vi "Limit ILC Voltage.vi"(8 "error in (no error)":errorcluster, 10 "Voltage in":dbl[unit], 11 "Limit ILC Voltage in":refnum<class "Limit ILC Voltage.lvclass">) -> (0 "error out":errorcluster, 2 "Voltage out":dbl[unit], 3 "Limit ILC Voltage out":refnum<class "Limit ILC Voltage.lvclass">)   [LabVIEW 2015, in "Limit ILC Voltage.lvclass"]
uses:
  Limit ILC Voltage.lvclass
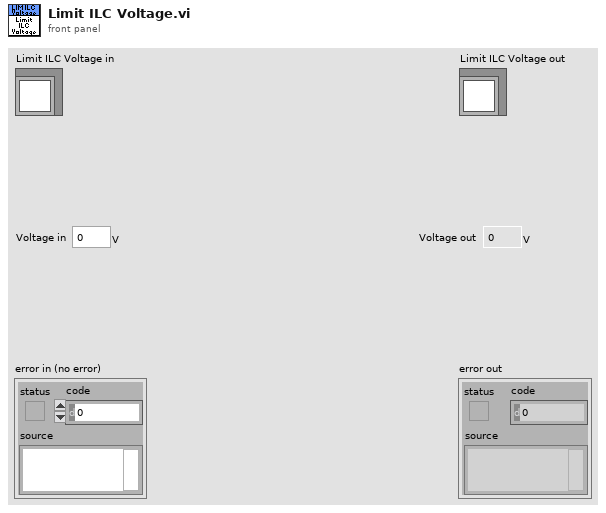
[diagram p1: front panel]
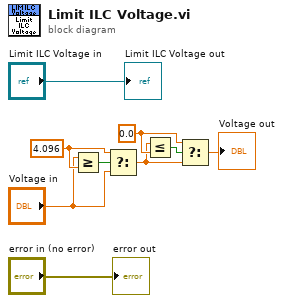
[diagram p0: block diagram]
diagram:
  w3 = dbl[unit] 0.0 ("y")
  w6 = dbl[unit] 4.096 ("y")
  n1 = Greater Or Equal?(x="Voltage in", y=w6) -> (x >= y?=w7:bool)
  n2 = Select(t=w6, s=w7, f="Voltage in") -> (s? t:f=w2:dbl[unit])
  n3 = Less Or Equal?(x=w2, y=w3) -> (x <= y?=w4:bool)
  n4 = Select(t=w3, s=w4, f=w2) -> (s? t:f=→"Voltage out":dbl[unit])
  "error out" <- "error in (no error)"
  "Limit ILC Voltage out" <- "Limit ILC Voltage in"
